vi "BlueSerializationProviderDependencyLinker.vi"   [LabVIEW 2019]
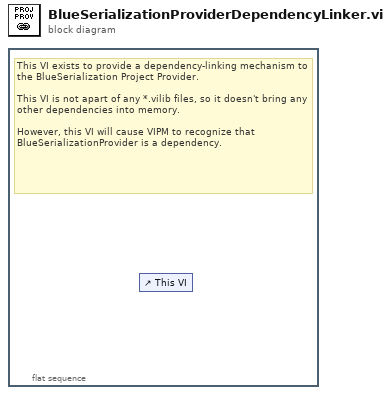
[diagram p0: block diagram]
diagram:
  n1 = flat-sequence {
    frame #0 {
      # "This VI exists to provide a dependency-linking mechanism to the BlueSerialization Project Provider.\n\nThis VI is not apart of any *.vilib files, so it doesn't bring any other dependencies into memory.\n\nHowever, this VI will cause VIPM to recognize that BlueSerializationProvider is a dependency."
      n2 = control-ref of="This VI"() -> ()  [unwired: 1 out]
    }
  }
